vi "evaluate_dependent_vars.vi"(7 "current independent variable values":dbl[](array[numeric]), 8 "error in (no error)":errorcluster, 9 "dependent variable equations":string[](array[string]), 10 "dependent variable names":string[](array[string]), 11 "independent variable names":string[](array[string])) -> (0 "error out":errorcluster, 1 "dependent variable results":dbl[](array[numeric]), 2 "current all variable values":dbl[](array[numeric]), 3 "all variable names":string[](array[string]))   [LabVIEW 2013]
uses:
  <vilib>/gmath/NI_Gmath.lvlib
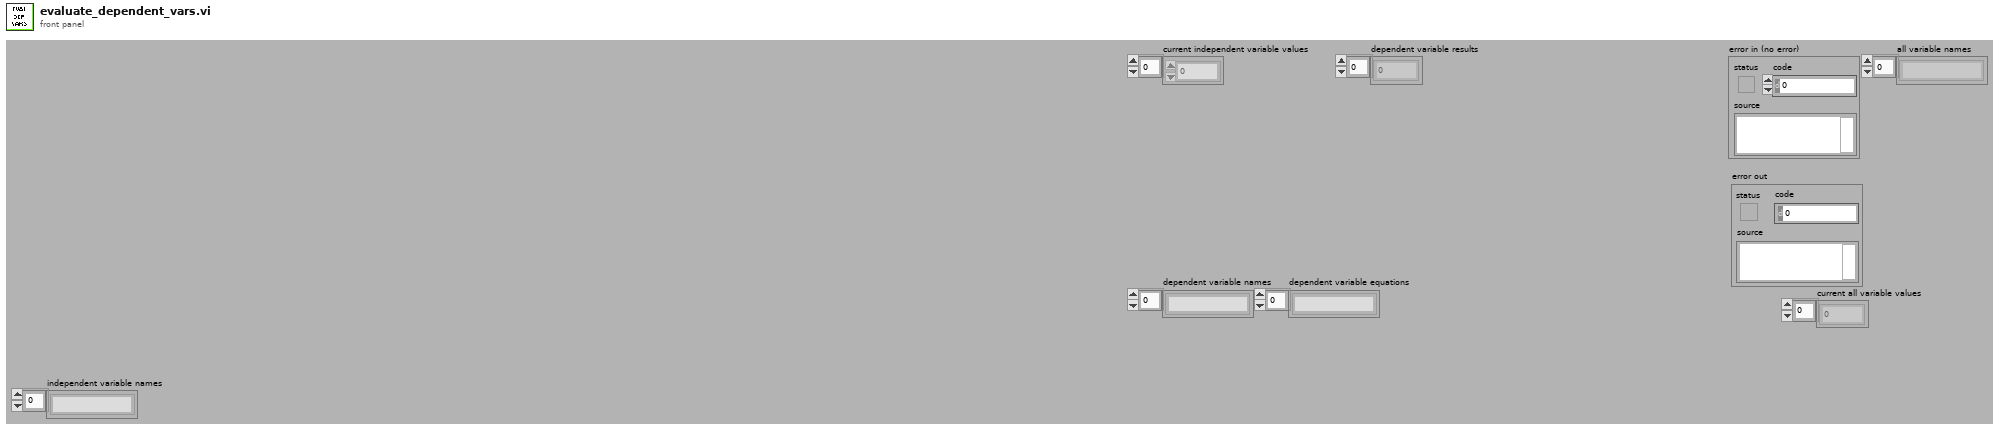
[diagram p1: front panel]
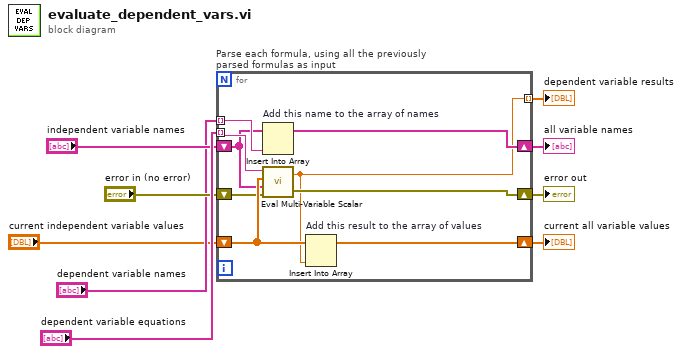
[diagram p0: block diagram]
diagram:
  n1 = for "Parse each formula, using all the previously parsed formulas as input" {
    tunnel: "dependent variable equations" -> [w18] mode=indexing
    shift-right: [w17] -> w9
    shift-left: "current independent variable values" -> [w16]
    shift-right: [w14] -> w6
    shift-left: "error in (no error)" -> [w15]
    shift-right: [w12] -> w5
    shift-left: "independent variable names" -> [w11]
    tunnel: "dependent variable names" -> [w13] mode=indexing
    tunnel: [w10] -> w1 mode=indexing
    n2 = Insert Into Array "Add this name to the array of names"(array=w11, new element=w13) -> (w12:string[])  [unwired: 1 in]
    n3 = call <vilib>:"Eval Multi-Variable Scalar.vi"("error in (no error)"=w15, "Variables"=w11, "X Values"=w16, "formula"=w18) -> ("error out"=w14:errorcluster, "y value"=w10:dbl)
    n4 = Insert Into Array "Add this result to the array of values"(array=w16, new element=w10) -> (w17:dbl[])  [unwired: 1 in]
  }
  "error out" <- w6
  "current all variable values" <- w9
  "all variable names" <- w5
  "dependent variable results" <- w1
